vi "Index Array Elements - refnum.vi"(4 "indices (none)":i32[](array[numeric])=[3, 5, 4], 7 "1D Array":refnum<vi>[](array[refnum])) -> (0 "output array":refnum<vi>[](array[refnum]))   [LabVIEW 2020]
doc: "Returns the elements of a 1-dimension array at indices. This is a list-based version of the built-in \"Index Array\"."
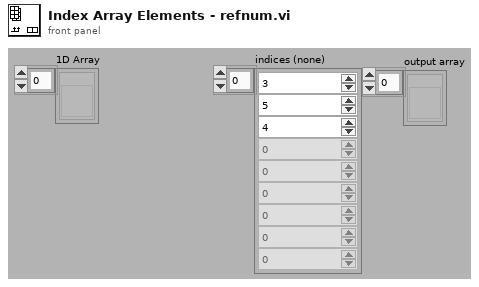
[diagram p1: front panel]
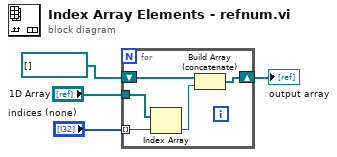
[diagram p0: block diagram]
diagram:
  n1 = for {
    shift-right: [w5] -> w3
    shift-left: refnum<vi>[] [] ("output array 2") -> [w7]
    tunnel: "indices (none)" -> [w8] mode=indexing
    tunnel: "1D Array" -> [w9]
    n2 = Index Array(array=w9, index=w8) -> (element=w6:refnum<vi>)
    n3 = Build Array (concatenate)(w7, w6) -> (w5:refnum<vi>[])
  }
  "output array" <- w3
